vi "Make Digital I-O Invert Arrays.vi"(8 "CalDataIn":T1(array[cluster])=[{"PageTitle"="SCXI-1520 Module 10 AIN", "NumLines"=8, "ChlNum"=["0", "1", "2", "3", "4", "5", "6", "7"], "ChlDesc"=["GBX Lube Pump Load Delta-P", "Fuel Pump Load Delta-P", "Generator #1 Load Delta-P", "Generator #2 Load Delta-P", "Hydraulic Pump Load Delta-P", "Gearbox Internal Pressure", "Gearbox Lube System Pressure", "Gearbox Air In Pressure"], "ChlUnits"=["psid", "psid", "psid", "psid", "psid", "psi", "psi", "psi"], "ChlZero"=[0.0, 0.0, 0.0, 0.0, 0.0, 0.0, 0.0, 0.0], "ChlFactor"=[100.0, 100.0, 100.0, 100.0, 100.0, 100.0, 100.0, 100.0], "ChlConfig"=[3, 3, 3, 3, 3, 3, 3, 3]}, {"PageTitle"="SCXI-1125 Module 7 AIN", "NumLines"=8, "ChlNum"=["0", "1", "2", "3", "4", "5", "6", "7"], "ChlDesc"=["T/S Speed", "T/S Flow", "GBX Oil Lube Pump In Flow", "Breather Exit Pressure", "Lube Jet #2 Pressure", "<spare>", "<spare>", "<spare>"], "ChlUnits"=["krpm", "gpm", "gpm", "psi", "psi", "<none>", "<none>", "<none>"], "ChlZero"=[0.0, 0.0, 0.0, 0.0, 0.0, 0.0, 0.0, 0.0], "ChlFactor"=[100.0, 100.0, 100.0, 100.0, 100.0, 1.0, 1.0, 1.0], "ChlConfig"=[3, 3, 3, 3, 3, 3, 3, 3]}, {"PageTitle"="SCXI-1102 Chls 0-15 AIN", "NumLines"=16, "ChlNum"=["0", "1", "2", "3", "4", "5", "6", "7", "8", "9", "10", "11", "12", "13", "14", "15"], "ChlDesc"=["Bevel Gbx Sump Oil Temperature", "Bevel Gbx Lube Out Temperature", "Bevel Gbx Hxg Water Out Temp", "Bevel Gbx Water Out Temperature", "Bevel Gbx Top Ball Bearing Temp", "Bevel Gbx Internal Bearing Temp", "Bevel Gbx Forward Bearing Temp", "T/S Lube Sys Hxg Water Out Temp", "Gbx Oil In Temperature", "Gbx Oil Out Temperature", "Gbx Air In Temperature", "Gbx Air Out Temperature", "Gbx Hydraulic Reservoir Temp", "Gbx Hxg Water Out Temperature", "T/S Lube System In Temperature", "T/S Lube System Scavenge Temp"], "ChlUnits"=["Deg-F", "Deg-F", "Deg-F", "Deg-F", "Deg-F", "Deg-F", "Deg-F", "Deg-F", "Deg-F", "Deg-F", "Deg-F", "Deg-F", "Deg-F", "Deg-F", "Deg-F", "Deg-F"], "ChlZero"=[0.0, 0.0, 0.0, 0.0, 0.0, 0.0, 0.0, 0.0, 0.0, 0.0, 0.0, 0.0, 0.0, 0.0, 0.0, 0.0], "ChlFactor"=[1.0, 1.0, 1.0, 1.0, 1.0, 1.0, 1.0, 1.0, 1.0, 1.0, 1.0, 1.0, 1.0, 1.0, 1.0, 1.0], "ChlConfig"=[3, 3, 3, 3, 3, 3, 3, 3, 3, 3, 3, 3, 3, 3, 3, 3]}, {"PageTitle"="SCXI-1102 Chls 16-31 AIN", "NumLines"=16, "ChlNum"=["16", "17", "18", "19", "20", "21", "22", "23", "24", "25", "26", "27", "28", "29", "30", "31"], "ChlDesc"=["Lube Pump AFT Roller Brg Temp", "Super Charge Reservoir Temp", "Boost Pump Lube In Temperature", "Load Pump Reservoir Temp", "Case Flow Supply Temperature", "Water In Temperature", "Recirc Rsvr Hxg Water Out Temp", "Hydraulic Load Water Out Temp", "H/S S/I Aft Bearing Temp", "<spare>", "<spare>", "<spare>", "<spare>", "<spare>", "<spare>", "<spare>"], "ChlUnits"=["Deg-F", "Deg-F", "Deg-F", "Deg-F", "Deg-F", "Deg-F", "Deg-F", "Deg-F", "Deg-F", "<none>", "<none>", "<none>", "<none>", "<none>", "<none>", "<none>"], "ChlZero"=[0.0, 0.0, 0.0, 0.0, 0.0, 0.0, 0.0, 0.0, 0.0, 0.0, 0.0, 0.0, 0.0, 0.0, 0.0, 0.0], "ChlFactor"=[1.0, 1.0, 1.0, 1.0, 1.0, 1.0, 1.0, 1.0, 1.0, 1.0, 1.0, 1.0, 1.0, 1.0, 1.0, 1.0], "ChlConfig"=[3, 3, 3, 3, 3, 3, 3, 3, 3, 3, 3, 3, 3, 3, 3, 3]}, {"PageTitle"="SCXI-1124 Module 5 AOUT", "NumLines"=6, "ChlNum"=["0", "1", "2", "3", "4", "5"], "ChlDesc"=["Speed", "GBX Oil Lube Pump In Flow", "GBX HX Water Flow", "GBX Oil Temperature", "<spare>", "<spare>"], "ChlUnits"=["rpm", "gpm", "gpm", "Deg-F", "<none>", "<none>"], "ChlZero"=[0.0, 0.0, 0.0, 0.0, 0.0, 0.0], "ChlFactor"=[100.0, 100.0, 100.0, 100.0, 1.0, 1.0], "ChlConfig"=[2, 2, 2, 2, 2, 2]}, {"PageTitle"="SCXI-1124 Module 6 AOUT", "NumLines"=6, "ChlNum"=["0", "1", "2", "3", "4", "5"], "ChlDesc"=["GBX Oil Lube Pump Load Delta-P", "Fuel Pump Load Delta-P", "Generator #1 Load Delta-P", "Generator #1 Load Delta-P", "Hydraulic Pump Load Delta-P", "<spare>"], "ChlUnits"=["psid", "psid", "psid", "psid", "psid", "<none>"], "ChlZero"=[0.0, 0.0, 0.0, 0.0, 0.0, 0.0], "ChlFactor"=[100.0, 100.0, 100.0, 100.0, 100.0, 1.0], "ChlConfig"=[2, 2, 2, 2, 2, 2]}, {"PageTitle"="SCXI-1162HV Chls 0-15 DIN", "NumLines"=16, "ChlNum"=["0", "1", "2", "3", "4", "5", "6", "7", "8", "9", "10", "11", "12", "13", "14", "15"], "ChlDesc"=["Emergency Switch", "Bevel Level Filter Delta-P Switch", "Bevel GBX Reservoir Level", "Bevel GBX Lube Over Pressure", "Bevel GBX Lube Under Pressure", "Bevel GBX Scav Pump Motor Fbk", "Bevel GBX Lube Pump Motor Fbk", "GBX Lube Reservoir Level", "GBX Lube Rsvr Circ Pump Motor", "T/S Lube System Pressure", "T/S Lube System Scav Motor Fbk", "Air In Pressure", "Water In Pressure", "Load Super Charge Pressure", "Boost Pump Reservoir Level", "Lube System Pump Motor Fbk"], "ChlUnits"=["DIN", "DIN", "DIN", "DIN", "DIN", "DIN", "DIN", "DIN", "DIN", "DIN", "DIN", "DIN", "DIN", "DIN", "DIN", "DIN"], "ChlZero"=[0.0, 0.0, 0.0, 0.0, 0.0, 0.0, 0.0, 0.0, 0.0, 0.0, 0.0, 0.0, 0.0, 0.0, 0.0, 0.0], "ChlFactor"=[1.0, 1.0, 1.0, 1.0, 1.0, 1.0, 1.0, 1.0, 1.0, 1.0, 1.0, 1.0, 1.0, 1.0, 1.0, 1.0], "ChlConfig"=[11, 11, 11, 11, 11, 11, 11, 11, 11, 11, 11, 11, 11, 11, 11, 11]}, {"PageTitle"="SCXI-1162HV Chls 16-31 DIN", "NumLines"=16, "ChlNum"=["16", "17", "18", "19", "20", "21", "22", "23", "24", "25", "26", "27", "28", "29", "30", "31"], "ChlDesc"=["<spare>", "<spare>", "<spare>", "<spare>", "<spare>", "<spare>", "<spare>", "<spare>", "<spare>", "<spare>", "<spare>", "<spare>", "<spare>", "<spare>", "<spare>", "<spare>"], "ChlUnits"=["DIN", "DIN", "DIN", "DIN", "DIN", "DIN", "DIN", "DIN", "DIN", "DIN", "DIN", "DIN", "DIN", "DIN", "DIN", "DIN"], "ChlZero"=[0.0, 0.0, 0.0, 0.0, 0.0, 0.0, 0.0, 0.0, 0.0, 0.0, 0.0, 0.0, 0.0, 0.0, 0.0, 0.0], "ChlFactor"=[1.0, 1.0, 1.0, 1.0, 1.0, 1.0, 1.0, 1.0, 1.0, 1.0, 1.0, 1.0, 1.0, 1.0, 1.0, 1.0], "ChlConfig"=[11, 11, 11, 11, 11, 11, 11, 11, 11, 11, 11, 11, 11, 11, 11, 11]}, {"PageTitle"="SCXI-1163R Chls 0-15 DOUT", "NumLines"=16, "ChlNum"=["0", "1", "2", "3", "4", "5", "6", "7", "8", "9", "10", "11", "12", "13", "14", "15"], "ChlDesc"=["DC Motor Start Relay", "DC Motor Stop Relay", "Bevel GBX Scavenge Pump", "Bevel GBX Lube Pump", "GBX Lube Rsvr Circulation Pump", "GBX Oil Lube Pump", "GBX Lube System Scavenge Pump", "T/S Lube System Scavenge Pump", "T/S Lube System Pump", "Load Boost Pump", "Load Pump Case Drain Pump", "Water Pump", "<spare>", "<spare>", "<spare>", "<spare>"], "ChlUnits"=["DOUT", "DOUT", "DOUT", "DOUT", "DOUT", "DOUT", "DOUT", "DOUT", "DOUT", "DOUT", "DOUT", "DOUT", "DOUT", "DOUT", "DOUT", "DOUT"], "ChlZero"=[0.0, 0.0, 0.0, 0.0, 0.0, 0.0, 0.0, 0.0, 0.0, 0.0, 0.0, 0.0, 0.0, 0.0, 0.0, 0.0], "ChlFactor"=[1.0, 1.0, 1.0, 1.0, 1.0, 1.0, 1.0, 1.0, 1.0, 1.0, 1.0, 1.0, 1.0, 1.0, 1.0, 1.0], "ChlConfig"=[12, 12, 12, 12, 12, 12, 12, 12, 12, 12, 12, 12, 12, 12, 12, 12]}, {"PageTitle"="SCXI-1163R Chls 15-31 DOUT", "NumLines"=16, "ChlNum"=["16", "17", "18", "19", "20", "21", "22", "23", "24", "25", "26", "27", "28", "29", "30", "31"], "ChlDesc"=["<spare>", "<spare>", "<spare>", "<spare>", "<spare>", "<spare>", "<spare>", "<spare>", "<spare>", "<spare>", "<spare>", "<spare>", "<spare>", "<spare>", "<spare>", "<spare>"], "ChlUnits"=["DOUT", "DOUT", "DOUT", "DOUT", "DOUT", "DOUT", "DOUT", "DOUT", "DOUT", "DOUT", "DOUT", "DOUT", "DOUT", "DOUT", " DOUT", "DOUT"], "ChlZero"=[0.0, 0.0, 0.0, 0.0, 0.0, 0.0, 0.0, 0.0, 0.0, 0.0, 0.0, 0.0, 0.0, 0.0, 0.0, 0.0], "ChlFactor"=[1.0, 1.0, 1.0, 1.0, 1.0, 1.0, 1.0, 1.0, 1.0, 1.0, 1.0, 1.0, 1.0, 1.0, 1.0, 1.0], "ChlConfig"=[12, 12, 12, 12, 12, 12, 12, 12, 12, 12, 12, 12, 12, 12, 12, 12]}] {"ChlFactor" format="%.3f"; "ChlZero" format="%.3f"}, 10 "InvDins":bool, 11 "InvDouts":bool) -> (0 "DIO-Inv":bool[][](array[boolean]), 1 "DoutInit":i32[](array[numeric]), 2 "NumDoutPages":i32, 3 "NumDinPages":i32, 4 "DoutInv (2D)":bool[][](array[boolean]), 5 "DinInv (2D)":bool[][](array[boolean]), 6 "DoutInv (1D)":bool[](array[boolean]), 7 "DinInv (1D)":bool[](array[boolean]))   [LabVIEW 2013]
panel:
  in  "Lines/Page":i32=8
  in  "NumPages":i32=10
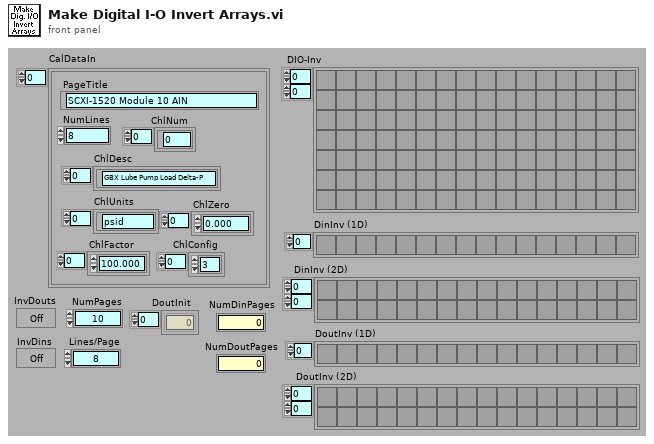
[diagram p1: front panel]
types:
  T1 = cluster{"PageTitle":string, "NumLines":i32, "ChlNum":string[], "ChlDesc":string[], "ChlUnits":string[], "ChlZero":sgl[], "ChlFactor":sgl[], "ChlConfig":u16[]}[]
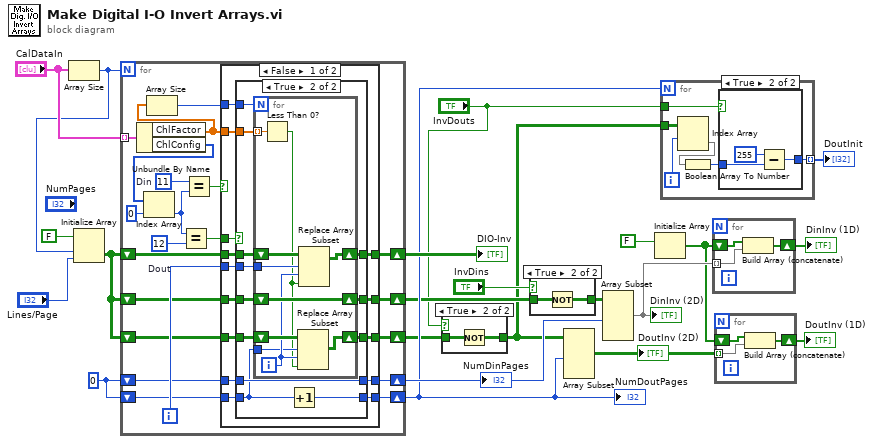
[diagram p0: block diagram]
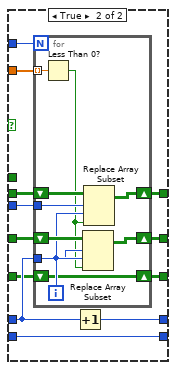
[diagram p6: hidden frame]
diagram:
  w21 = 0
  n1 = Array Size(array="CalDataIn") -> (size(s)=w15:i32)
  n2 = Initialize Array(FALSE, w15, "Lines/Page") -> (w18:bool[][])
  n3 = for {
    N: w15 -> [_]
    tunnel: "CalDataIn" -> [w43] mode=indexing
    shift-right: [w30] -> w13
    shift-left: w21 -> [w31]
    shift-right: [w29] -> w12
    shift-left: w21 -> [w28]
    shift-right: [w33] -> w19
    shift-left: w18 -> [w34]
    shift-right: [w26] -> w6
    shift-left: w18 -> [w27]
    shift-right: [w24] -> w3
    shift-left: w18 -> [w25]
    i -> [w32]
    w38 = u16 11  # Din
    w40 = u16 12  # Dout
    n4 = Unbundle By Name(w43) -> ("ChlFactor"=w23:sgl[], "ChlConfig"=w41:u16[])
    n5 = Index Array(array=w41, index=0 ("Index")) -> (element=w39:u16)
    n6 = Array Size(array=w23) -> (size(s)=w35:i32)
    n7 = Equal?(x=w39, y=w40) -> (x = y?=w36:bool)
    n8 = Equal?(x=w38, y=w39) -> (x = y?=w37:bool)
    n9 = case shown="False" w37 {
      tunnel: w36 -> [w57 _]
      tunnel: w35 -> [w52 w96]
      tunnel: w23 -> [w48 w95]
      tunnel: w34 -> [w50 w91]
      tunnel: [w49 w90] -> w33
      tunnel: w32 -> [w51 w94]
      tunnel: w31 -> [w56 w88]
      tunnel: [w55 w93] -> w30
      tunnel: [w53 w92] -> w29
      tunnel: w28 -> [w54 w92]
      tunnel: w27 -> [w47 w89]
      tunnel: [w46 w87] -> w26
      tunnel: w25 -> [w45 w86]
      tunnel: [w44 w85] -> w24
      frame False {
        n10 = case shown="True" w57 {
          tunnel: w56 -> [w62 w74]
          tunnel: [w62 w74] -> w55
          tunnel: w54 -> [w61 w64]
          tunnel: [w61 w73] -> w53
          tunnel: w52 -> [_ w72]
          tunnel: w51 -> [_ w71]
          tunnel: w50 -> [w60 w69]
          tunnel: [w60 w68] -> w49
          tunnel: w48 -> [_ w70]
          tunnel: w47 -> [w59 w67]
          tunnel: [w59 w66] -> w46
          tunnel: w45 -> [w58 w65]
          tunnel: [w58 w63] -> w44
          frame False {
          }
          frame True {
            n11 = for {
              N: w72 -> [_]
              tunnel: w71 -> [w81]
              tunnel: w70 -> [w84] mode=indexing
              shift-right: [w82] -> w68
              shift-left: w69 -> [w83]
              shift-right: [w80] -> w66
              shift-left: w67 -> [w80]
              shift-right: [w78] -> w63
              shift-left: w65 -> [w79]
              tunnel: w64 -> [w76]
              i -> [w77]
              n12 = Less Than 0?(x=w84) -> (x < 0?=w75:bool)
              n13 = Replace Array Subset(array=w79, new element=w75, index (row)=w76, index (col)=w77) -> (w78:bool[][])
              n14 = Replace Array Subset(array=w83, new element=w75, index (row)=w81, index (col)=w77) -> (w82:bool[][])
            }
            n15 = Increment(x=w64) -> (x+1=w73:i32)
          }
        }
      }
      frame True {
        n16 = for {
          N: w96 -> [_]
          tunnel: w95 -> [w106] mode=indexing
          tunnel: w94 -> [w103]
          shift-right: [w104] -> w90
          shift-left: w91 -> [w105]
          shift-right: [w99] -> w87
          shift-left: w89 -> [w102]
          shift-right: [w98] -> w85
          shift-left: w86 -> [w98]
          tunnel: w88 -> [w100]
          i -> [w101]
          n17 = Less Than 0?(x=w106) -> (x < 0?=w97:bool)
          n18 = Replace Array Subset(array=w102, new element=w97, index (row)=w100, index (col)=w101) -> (w99:bool[][])
          n19 = Replace Array Subset(array=w105, new element=w97, index (row)=w103, index (col)=w101) -> (w104:bool[][])
        }
        n20 = Increment(x=w88) -> (x+1=w93:i32)
      }
    }
  }
  "NumDoutPages" <- w12
  "NumDinPages" <- w13
  "DIO-Inv" <- w19
  n21 = case shown="True" "InvDouts" {
    tunnel: w3 -> [w107 w109]
    tunnel: [w107 w108] -> w2
    frame False {
    }
    frame True {
      n22 = Not(x=w109) -> (.not. x?=w108:bool[][])
    }
  }
  n23 = case shown="True" "InvDins" {
    tunnel: w6 -> [w110 w112]
    tunnel: [w110 w111] -> w5
    frame False {
    }
    frame True {
      n24 = Not(x=w112) -> (.not. x?=w111:bool[][])
    }
  }
  n25 = Array Subset(array=w2, length (row)=w12) -> (w9:bool[][])  [unwired: 3 in]
  "DoutInv (2D)" <- w9
  n26 = Array Subset(array=w5, length (row)=w13) -> (w14:bool[][])  [unwired: 3 in]
  "DinInv (2D)" <- w14
  n27 = Initialize Array(FALSE) -> (w8:bool[])  [unwired: 1 in]
  n28 = for {
    N: w12 -> [_]
    tunnel: w2 -> [w117]
    tunnel: [w114] -> w17 mode=indexing
    tunnel: "InvDouts" -> [w113]
    i -> [w118]
    n29 = Index Array(array=w117, index (row)=w118) -> (element=w116:bool[])  [unwired: 1 in]
    n30 = Boolean Array To Number(Boolean array=w116) -> (number=w115:u32)
    n31 = case shown="True" w113 {
      tunnel: w115 -> [w119 w122]
      tunnel: [w119 w120] -> w114
      frame False {
      }
      frame True {
        n32 = Subtract(x=u32 255, y=w122) -> (x-y=w120:u32)
      }
    }
  }
  "DoutInit" <- w17
  n33 = for {
    shift-right: [w123] -> w10
    shift-left: w8 -> [w124]
    tunnel: w14 -> [w125] mode=indexing
    n34 = Build Array (concatenate)(w124, w125) -> (w123:bool[])
  }
  "DinInv (1D)" <- w10
  n35 = for {
    shift-right: [w126] -> w7
    shift-left: w8 -> [w127]
    tunnel: w9 -> [w128] mode=indexing
    n36 = Build Array (concatenate)(w127, w128) -> (w126:bool[])
  }
  "DoutInv (1D)" <- w7
